vi "Get Rx Monitor Utilization.vi"() -> (3 "channel array":string[](array[string]))   [LabVIEW 2020, in "AIM ARINC 664 Scripting.lvlib"]
uses:
  AIM ARINC 664 Scripting.lvlib
  Constants.vi
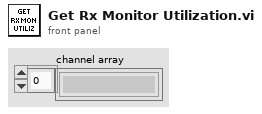
[diagram p1: front panel]
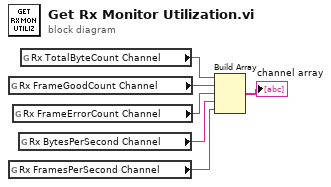
[diagram p0: block diagram]
diagram:
  n1 = global read "Constants.vi" "Rx FrameGoodCount Channel"() -> (w5:string)
  n2 = global read "Constants.vi" "Rx FramesPerSecond Channel"() -> (w2:string)
  n3 = global read "Constants.vi" "Rx FrameErrorCount Channel"() -> (w4:string)
  n4 = global read "Constants.vi" "Rx BytesPerSecond Channel"() -> (w3:string)
  n5 = global read "Constants.vi" "Rx TotalByteCount Channel"() -> (w6:string)
  n6 = Build Array(w6, w5, w4, w3, w2) -> (→"channel array":string[])
